vi "Img Update c Point.vi"(8 "error in (no error)":errorcluster, 11 "LF2R IDE in":refnum<class "Main Panel.lvclass">) -> (0 "error out":errorcluster, 3 "LF2R IDE out":refnum<class "Main Panel.lvclass">)   [LabVIEW 2018, in "Main Panel.lvlib" / "Main Panel.lvclass"]
uses:
  Main Panel.lvclass
  Image/Image Process.lvclass
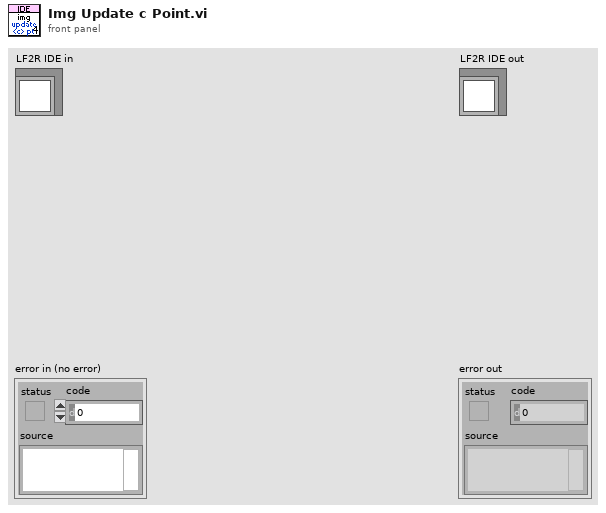
[diagram p1: front panel]
types:
  T1 = typedef "IMAQ Image.ctl" = refnum<image>
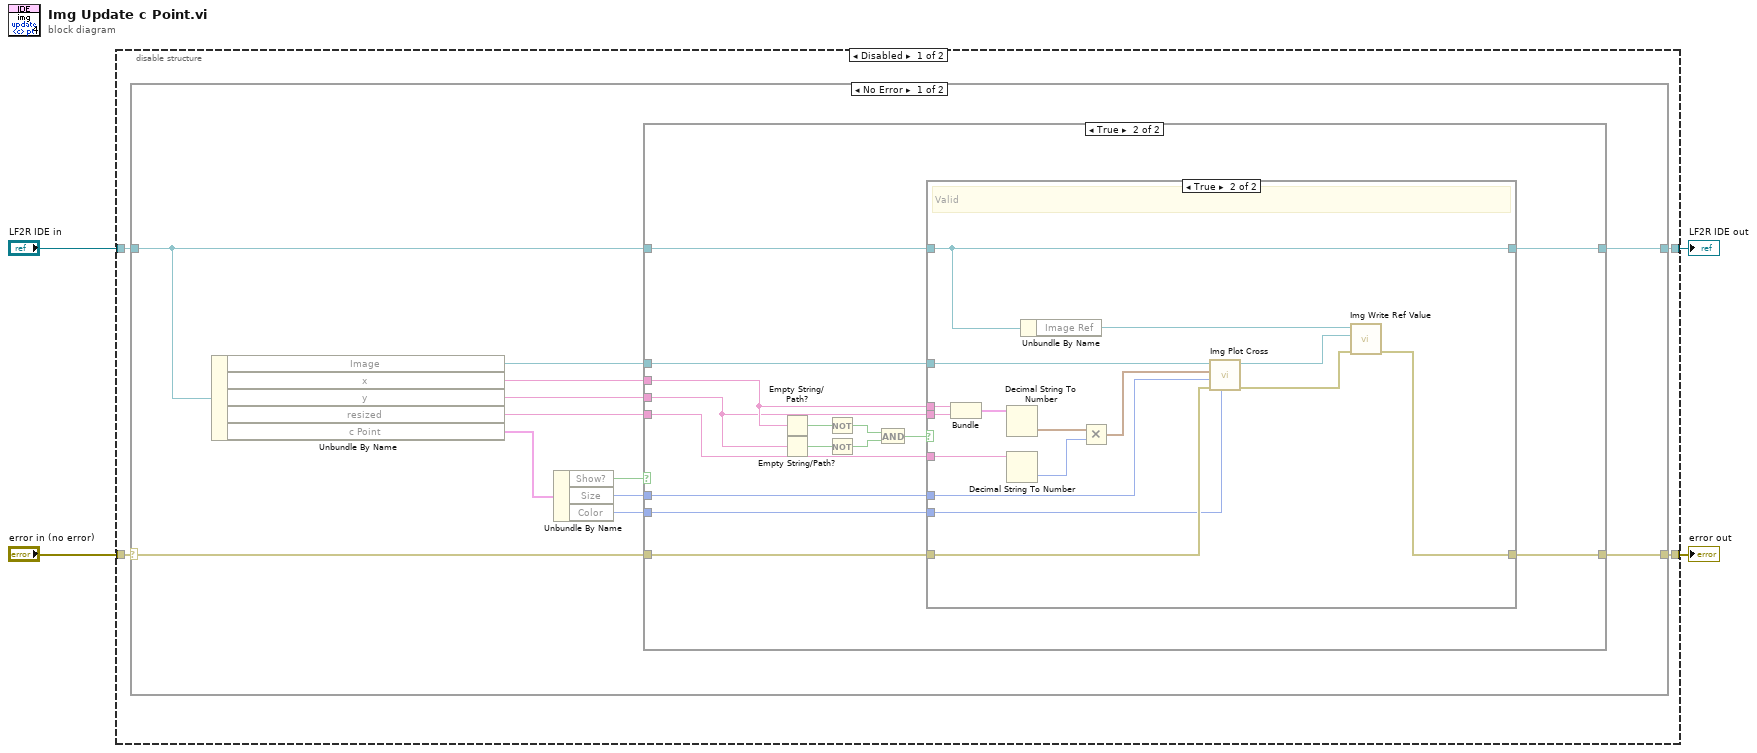
[diagram p0: block diagram]
diagram:
  n1 = disable-structure shown="Disabled" {
    disable-tunnel: "error in (no error)" -> [w8 w58]
    disable-tunnel: [w7 w58] -> w3
    disable-tunnel: "LF2R IDE in" -> [w6 w59]
    disable-tunnel: [w5 w59] -> w1
    frame Disabled {
      n2 = case shown="No Error" w8 {
        selector: w8 -> [w16 w57]
        tunnel: [w19 w57] -> w7
        tunnel: [w13 w56] -> w5
        tunnel: w6 -> [w20 w56]
        frame No Error {
          n3 = Unbundle By Name(w20) -> ("Image"=w17:T1, "x"=w15:string, "y"=w14:string, "resized"=w18:string, "c Point"=w12:cluster{"Size":i32, "Color":u32, "Show?":bool})
          n4 = Unbundle By Name(w12) -> ("Show?"=w11:bool, "Size"=w10:i32, "Color"=w9:u32)
          n5 = case shown="True" w11 {
            tunnel: w20 -> [w22 w37]
            tunnel: [w21 w36] -> w19
            tunnel: w18 -> [_ w35]
            tunnel: w17 -> [_ w34]
            tunnel: w16 -> [w21 w33]
            tunnel: w15 -> [_ w32]
            tunnel: w14 -> [_ w31]
            tunnel: [w22 w25] -> w13
            tunnel: w10 -> [_ w24]
            tunnel: w9 -> [_ w23]
            frame False {
            }
            frame True {
              n6 = Empty String/Path?(string/path=w32) -> (empty?=w30:bool)
              n7 = Empty String/Path?(string/path=w31) -> (empty?=w29:bool)
              n8 = Not(x=w30) -> (.not. x?=w28:bool)
              n9 = Not(x=w29) -> (.not. x?=w27:bool)
              n10 = And(x=w28, y=w27) -> (x .and. y?=w26:bool)
              n11 = case shown="True" w26 {
                tunnel: w37 -> [w39 w42]
                tunnel: [w38 w54] -> w36
                tunnel: w35 -> [_ w53]
                tunnel: w34 -> [_ w50]
                tunnel: w33 -> [w38 w48]
                tunnel: w32 -> [_ w45]
                tunnel: w31 -> [_ w44]
                tunnel: [w39 w42] -> w25
                tunnel: w24 -> [_ w41]
                tunnel: w23 -> [_ w40]
                frame False {
                  # "Invalid"
                }
                frame True {
                  # "Valid"
                  n12 = Bundle("x"=w45, "y"=w44) -> (w43:cluster{"x":string, "y":string})  [unwired: 1 in]
                  n13 = Decimal String To Number(string=w43) -> (number=w52:cluster{"x":i32, "y":i32})  [unwired: 2 in, 1 out]
                  n14 = Decimal String To Number(string=w53) -> (number=w51:i32)  [unwired: 2 in, 1 out]
                  n15 = Unbundle By Name(w42) -> ("Image Ref"=w55:refnum<vi>)
                  n16 = Multiply(x=w52, y=w51) -> (x*y=w49:cluster{"x":i32, "y":i32})
                  n17 = call "Img Plot Cross.vi"("Color"=w40, "error in (no error)"=w48, "size"=w41, "position"=w49, "Image In"=w50) -> ("error out"=w47:errorcluster, "Image Out"=w46:T1)  [unwired: 5 in]
                  n18 = call "Img Write Ref Value.vi"("error in (no error)"=w47, "Image"=w46, "Image Ref"=w55) -> ("error out"=w54:errorcluster)  [unwired: 8 in]
                }
              }
            }
          }
        }
        frame Error {
        }
      }
    }
    frame Enabled {
    }
  }
  "error out" <- w3
  "LF2R IDE out" <- w1
